vi "sendData.vi"(2 "error in":errorcluster, 3 "connection ID":refnum<k5>, 4 "DATA":string) -> (0 "error out":errorcluster, 1 "connection ID out":refnum<k5>)   [LabVIEW 2023]
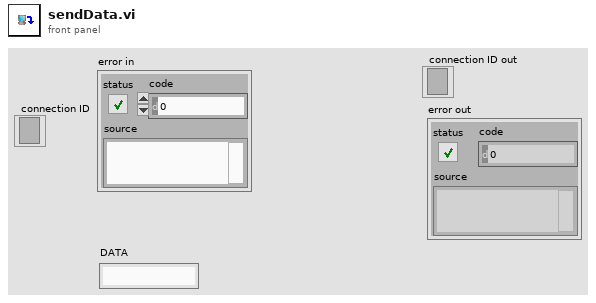
[diagram p1: front panel]
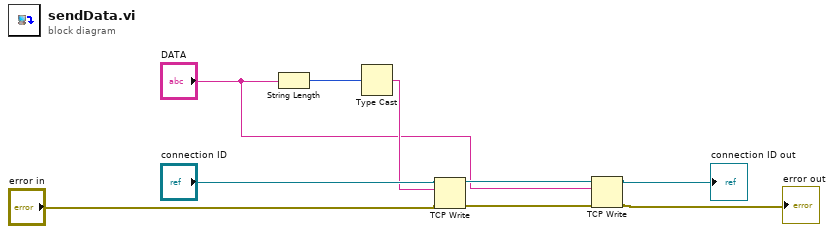
[diagram p0: block diagram]
diagram:
  n1 = String Length(string="DATA") -> (length=w3:i32)
  n2 = Type Cast(x=w3) -> (*(type *) &x=w2:string)  [unwired: 1 in]
  n3 = TCP Write(connection ID="connection ID", data in=w2, error in (no error)="error in") -> (connection ID out=w9:refnum<k5>, error out=w8:errorcluster)  [unwired: 1 in, 1 out]
  n4 = TCP Write(connection ID=w9, data in="DATA", error in (no error)=w8) -> (connection ID out=→"connection ID out":refnum<k5>, error out=→"error out":errorcluster)  [unwired: 1 in, 1 out]
